vi "Send Return Device IED_Status.vi"(5 "Message Type":refnum<class "Return Device IED_Status Msg.lvclass">, 7 "Message Priority (Normal)":T4=enum."Normal", 8 "error in (no error)":errorcluster, 10 "IED_Status":T1, 11 "Message Enqueuer":refnum<class "Message Enqueuer.lvclass">) -> (0 "error out":errorcluster, 3 "Message Enqueuer out":refnum<class "Message Enqueuer.lvclass">)   [LabVIEW 2016, in "Return Device IED_Status Msg.lvclass"]
doc: "This VI sends the message to an actor."
uses:
  Return Device IED_Status Msg.lvclass
  <vilib>/ActorFramework/Message Enqueuer/Message Enqueuer.lvclass
  <vilib>/ActorFramework/Message Enqueuer/Message Priority.ctl
  C:/Program Files (x86)/National Instruments/LabVIEW 2016/vi.lib/ActorFramework/Message/Message.lvclass
  <vilib>/ORNL/CSEISMIC DDS/CSEISMIC DDS Base/Data Types/IED_Status.ctl
  <vilib>/ORNL/CSEISMIC DDS/CSEISMIC DDS Base/Data Types/Controls/DeviceID.ctl
  <vilib>/ORNL/CSEISMIC DDS/CSEISMIC DDS Base/Data Types/Controls/Timestamp.ctl
  Return Device IED_Status Msg.lvclass/Return Device IED_Status Msg.ctl
  <vilib>/ActorFramework/Message Enqueuer/Message Enqueuer.lvclass/Message Enqueuer.ctl
  <vilib>/ActorFramework/Message Priority Queue/Priority Enqueue.vi
  <vilib>/ORNL/CSEISMIC DDS/CSEISMIC DDS Base/CSEISMIC DDS.lvclass
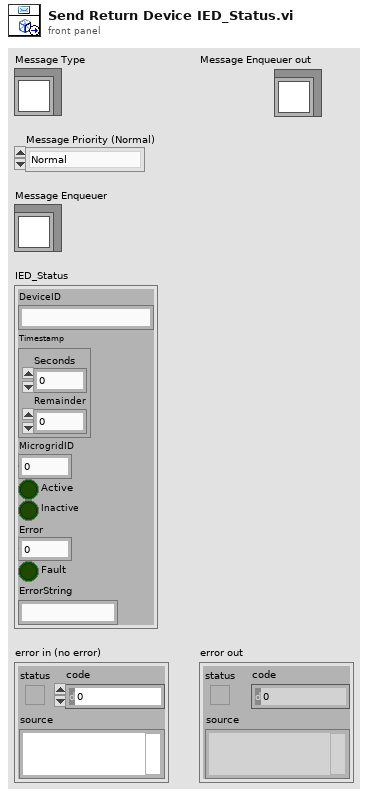
[diagram p1: front panel]
types:
  T1 = typedef "CSEISMIC DDS.lvlib/CSEISMIC DDS.lvclass/IED_Status.ctl" = cluster{"DeviceID":T2, "Timestamp":T3, "MicrogridID":u8, "Active":bool, "Inactive":bool, "Error":i32, "Fault":bool, "ErrorString":string}
  T2 = typedef "CSEISMIC DDS.lvlib/CSEISMIC DDS.lvclass/DeviceID.ctl" = string
  T3 = typedef "CSEISMIC DDS.lvlib/CSEISMIC DDS.lvclass/Timestamp.ctl" = cluster{"Seconds":u64, "Remainder":u64}
  T4 = typedef "Actor Framework.lvlib/Message Enqueuer.lvclass/Message Priority.ctl" = enum16{"Low", "Normal", "High"}
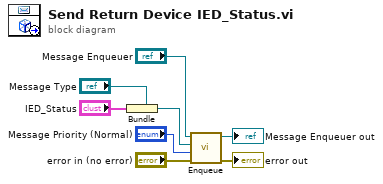
[diagram p0: block diagram]
diagram:
  n1 = Bundle(cluster="Message Type", "IED_Status") -> (w4:refnum<class "Return Device IED_Status Msg.lvclass">)
  n2 = call <vilib>:"Enqueue.vi"("error in (no error)"="error in (no error)", "Message Priority (Normal)"="Message Priority (Normal)", "Message"=w4, "Message Enqueuer in"="Message Enqueuer") -> ("error out"=→"error out":errorcluster, "Message Enqueuer out"=→"Message Enqueuer out":refnum<class "Message Enqueuer.lvclass">)  [unwired: 6 in]
